vi "Set Local Destination Directory.vi"(8 "error in (no error)":errorcluster, 10 "Directory path":path, 11 "BuildSpec in":refnum<vi>) -> (0 "error out":errorcluster, 3 "BuildSpec out":refnum<vi>)   [LabVIEW 2019, in "Project Sync Tools.lvclass"]
uses:
  Project Sync Tools.lvclass
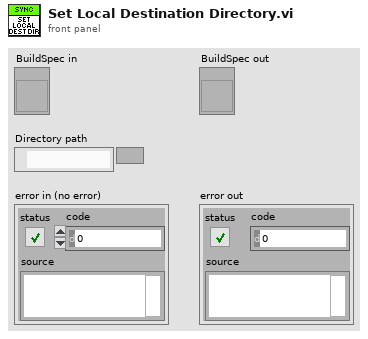
[diagram p1: front panel]
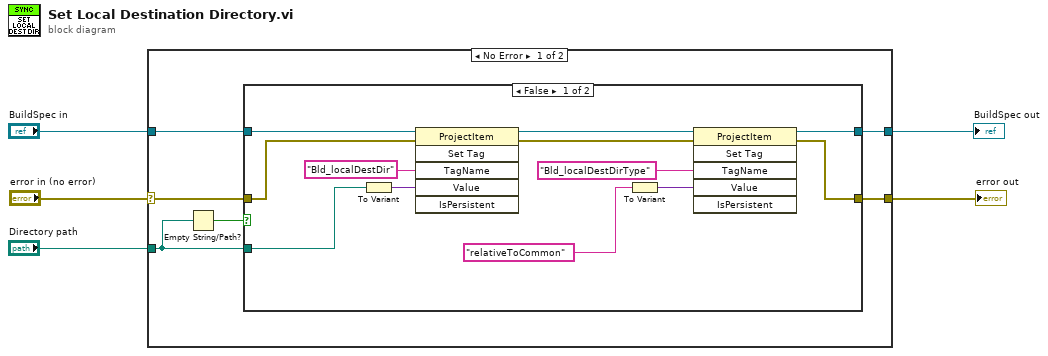
[diagram p0: block diagram]
diagram:
  n1 = case shown="No Error" "error in (no error)" {
    selector: "error in (no error)" -> [w8 w27]
    tunnel: "BuildSpec in" -> [w11 w26]
    tunnel: "Directory path" -> [w6 _]
    tunnel: [w10 w26] -> w3
    tunnel: [w9 w27] -> w2
    frame No Error {
      n2 = Empty String/Path?(string/path=w6) -> (empty?=w7:bool)
      n3 = case shown="False" w7 {
        tunnel: w11 -> [w23 w25]
        tunnel: w6 -> [w21 _]
        tunnel: [w17 w25] -> w10
        tunnel: [w16 w24] -> w9
        tunnel: w8 -> [w12 w24]
        frame False {
          n4 = To Variant(anything=w21) -> (Variant=w20:variant)
          n5 = invoke class="ProjectItem" method="Set Tag"(reference=w23, error in=w12, "TagName"="Bld_localDestDir" ("Tag Name"), "Value"=w20) -> (reference out=w19:refnum<vi>, error out=w18:errorcluster)  [unwired: 2 in, 4 out]
          n6 = To Variant(anything="relativeToCommon" ("Tag Name")) -> (Variant=w13:variant)
          n7 = invoke class="ProjectItem" method="Set Tag"(reference=w19, error in=w18, "TagName"="Bld_localDestDirType" ("Tag Name"), "Value"=w13) -> (reference out=w17:refnum<vi>, error out=w16:errorcluster)  [unwired: 2 in, 4 out]
        }
        frame True {
        }
      }
    }
    frame Error {
    }
  }
  "error out" <- w2
  "BuildSpec out" <- w3
